vi "query_outlets.vi"(11 "IP / Hostname":string="172.20.125.112") -> (0 "Return codes":i32[](array[numeric]), 3 "Switch status":bool[](array[boolean]))   [LabVIEW 2019]
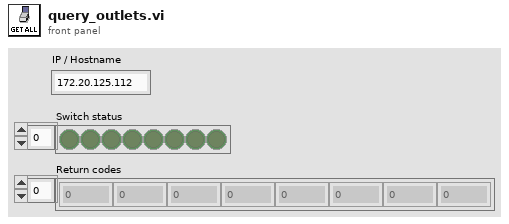
[diagram p1: front panel]
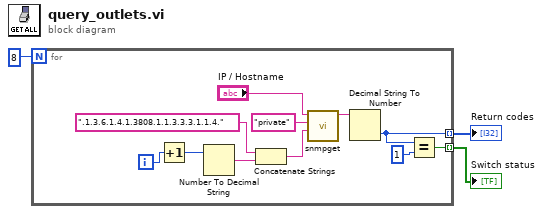
[diagram p0: block diagram]
diagram:
  n1 = for {
    N: 8 -> [_]
    tunnel: [w6] -> w2 mode=indexing
    tunnel: [w5] -> w1 mode=indexing
    i -> [w12]
    n2 = Increment(x=w12) -> (x+1=w11:i32)
    n3 = Number To Decimal String(number=w11) -> (decimal integer string=w9:string)  [unwired: 1 in]
    n4 = Concatenate Strings(".1.3.6.1.4.1.3808.1.1.3.3.3.1.1.4." ("OID"), w9) -> (w8:string)
    n5 = call "snmpget.vi"("OID"=w8, "community"="private", "IP / Hostname"="IP / Hostname") -> ("return"=w4:string)  [unwired: 7 in, 1 out]
    n6 = Decimal String To Number(string=w4) -> (number=w5:i32)  [unwired: 2 in, 1 out]
    n7 = Equal?(x=w5, y=1) -> (x = y?=w6:bool)
  }
  "Switch status" <- w2
  "Return codes" <- w1
